vi "read write configuration.vi"(7 "Enum":enum16{"Read", "Write"}(ring)=enum."Write", 8 "error in":errorcluster, 11 "Consumer Cluster in":T1={"This VI Ref"=refnum, "Test VI"=refnum, "Q Ref"=refnum, "UE"=refnum, "Data"=variant, "Timeout"=-1, "Path List[]"=[], "Status"="", "Counter"=0, "Config"={"Source Path"=path "", "Dest Path"=path "", "Log Path"=path "", "Move?"=FALSE, "Log?"=FALSE, "Scanners"=[], "Excude Folders"=[], "Jpg?"=FALSE, "Default path"=path "", "Extended?"=FALSE, "Mode"=enum."Move"}, "Total"=0, "Config Path"=path "", "exif info"={"Make"="Canon\u0000", "Model"="Canon PowerShot A495\u0000", "Orientation"=0, "Date"=timestamp(0 s since 1904-01-01), "Width"=0, "Height"=0, "Square?"=FALSE, "File Name"="Canon\u0000", "Extension"="Canon\u0000", "Valid?"=FALSE, "Path"=path "", "size"=0, "No Ext?"=FALSE, "prefix?"=FALSE, "String"="", "Name Type"=enum."Event Sufix"}, "app operation"=enum."Start", "Log Ref"=refnum, "Start Time"=0.0, "Pause Time"=0.0, "Argument?"=FALSE, "Argument path"=path "", "Identical"=FALSE, "File.lvclass"=refnum}) -> (0 "error out":errorcluster, 3 "cluster out":T1={"This VI Ref"=refnum, "Test VI"=refnum, "Q Ref"=refnum, "UE"=refnum, "Data"=variant, "Timeout"=-1, "Path List[]"=[], "Status"="", "Counter"=0, "Config"={"Source Path"=path "", "Dest Path"=path "", "Log Path"=path "", "Move?"=FALSE, "Log?"=FALSE, "Scanners"=[], "Excude Folders"=[], "Jpg?"=FALSE, "Default path"=path "", "Extended?"=FALSE, "Mode"=enum."Move"}, "Total"=0, "Config Path"=path "", "exif info"={"Make"="Canon\u0000", "Model"="Canon PowerShot A495\u0000", "Orientation"=0, "Date"=timestamp(0 s since 1904-01-01), "Width"=0, "Height"=0, "Square?"=FALSE, "File Name"="Canon\u0000", "Extension"="Canon\u0000", "Valid?"=FALSE, "Path"=path "", "size"=0, "No Ext?"=FALSE, "prefix?"=FALSE, "String"="", "Name Type"=enum."Event Sufix"}, "app operation"=enum."Start", "Log Ref"=refnum, "Start Time"=0.0, "Pause Time"=0.0, "Argument?"=FALSE, "Argument path"=path "", "Identical"=FALSE, "File.lvclass"=refnum})   [LabVIEW 2023, in "User Interface.lvlib"]
uses:
  User Interface.lvlib
  Controls/main consumer cluster.ctl
  File Classes/File/File.lvclass
  Controls/configuration cluster.ctl
  File Classes/Controls/exif data cluster.ctl
  File Classes/Controls/rename type enum.ctl
  Controls/app operation state enum.ctl
  File Classes/File Classes.lvlib
panel:
  # "Output Indicators"
  # "Input Controls"
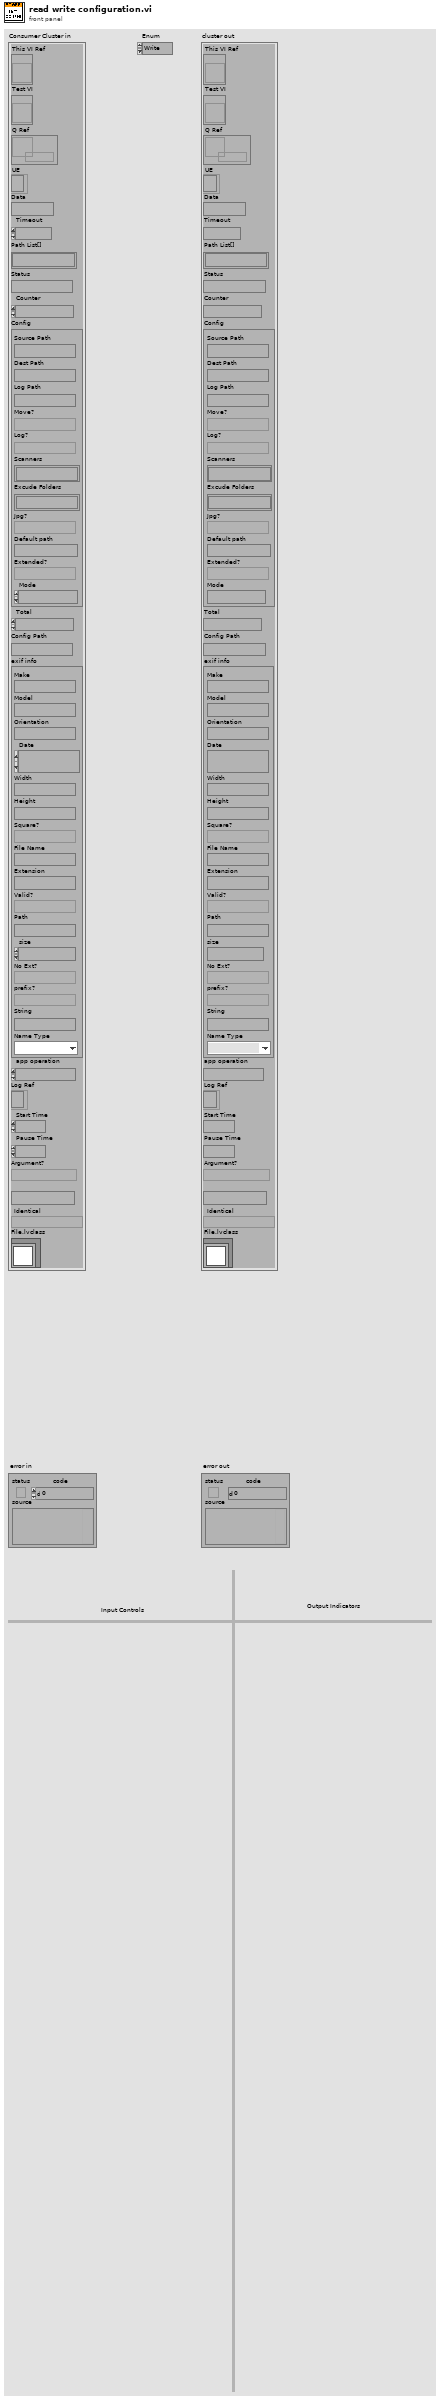
[diagram p1: front panel]
types:
  T1 = typedef "User Interface.lvlib/main consumer cluster.ctl" = cluster{"This VI Ref":refnum<vi>, "Test VI":refnum<vi>, "Q Ref":refnum<queue>, "UE":refnum<event-registration>, "Data":variant, "Timeout":i32, "Path List[]":path[], "Status":string, "Counter":i32, "Config":T2, "Total":i32, "Config Path":path, "exif info":T3, "app operation":T5, "Log Ref":refnum<file>, "Start Time":dbl, "Pause Time":dbl, "Argument?":bool, "Argument path":path, "Identical":bool, "File.lvclass":refnum<class "File.lvclass">}
  T2 = typedef "User Interface.lvlib/configuration cluster.ctl" = cluster{"Source Path":path, "Dest Path":path, "Log Path":path, "Move?":bool, "Log?":bool, "Scanners":string[], "Excude Folders":string[], "Jpg?":bool, "Default path":path, "Extended?":bool, "Mode":enum16{"Copy (Default)", "Move", "Rename"}}
  T3 = typedef "File Classes.lvlib/exif data cluster.ctl" = cluster{"Make":string, "Model":string, "Orientation":u16, "Date":timestamp, "Width":u16, "Height":u16, "Square?":bool, "File Name":string, "Extension":string, "Valid?":bool, "Path":path, "size":i64, "No Ext?":bool, "prefix?":bool, "String":string, "Name Type":T4}
  T4 = typedef "File Classes.lvlib/rename type enum.ctl" = enum16{"Date & Time (Default)", "Model Sufix", "Event Sufix", "Model & Event Sufix"}
  T5 = typedef "User Interface.lvlib/app operation state enum.ctl" = enum16{"Start", "Stop", "Pause", "Resume"}
  T6 = enum16{"open", "replace", "create", "open or create", "replace or create", "replace or create with confirmation"}
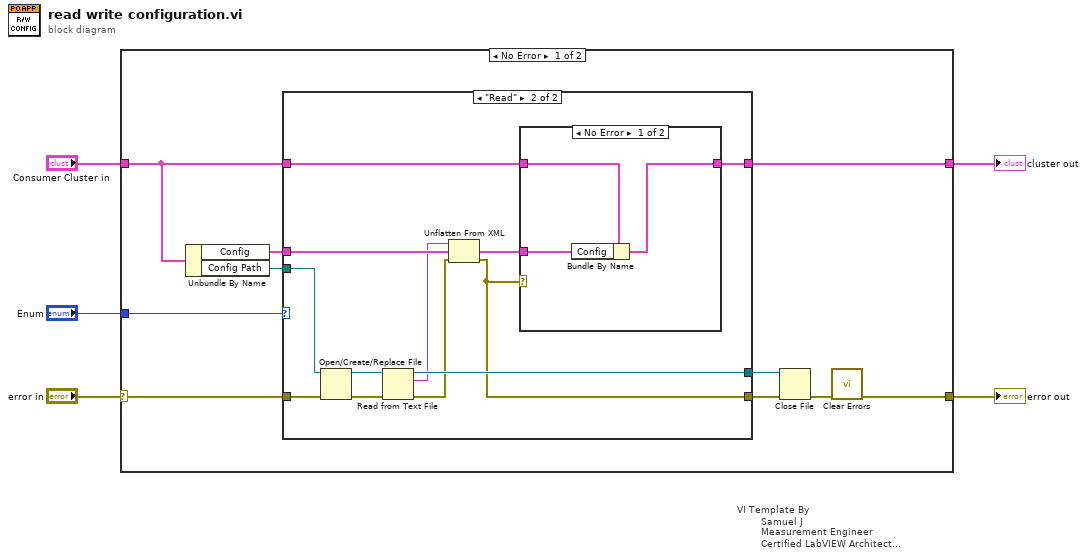
[diagram p0: block diagram]
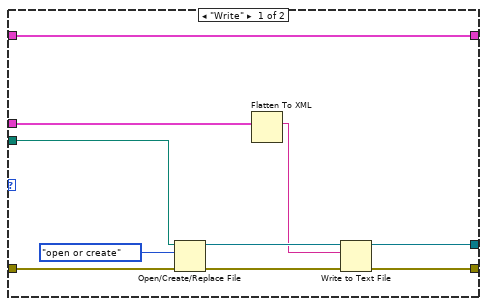
[diagram p2: hidden frame]
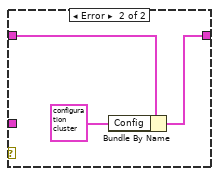
[diagram p3: hidden frame]
diagram:
  n1 = case "VI Template By\n        Samuel J\n        Measurement Engineer\n        Certified LabVIEW Architect\n        Vestas Technology R&D Chennai" shown="No Error" "error in" {
    selector: "error in" -> [w12 w45]
    tunnel: [w6 w45] -> w4
    tunnel: [w10 w44] -> w2
    tunnel: "Consumer Cluster in" -> [w9 w44]
    tunnel: "Enum" -> [w7 _]
    frame No Error {
      n2 = Unbundle By Name(w9) -> ("Config"=w13:T2, "Config Path"=w8:path)
      n3 = case shown="\"Read\"" w7 {
        tunnel: [w24 w36] -> w15
        tunnel: [w22 w26] -> w14
        tunnel: w13 -> [w21 w32]
        tunnel: w12 -> [w19 w34]
        tunnel: [w18 w28] -> w10
        tunnel: w9 -> [w18 w29]
        tunnel: w8 -> [w16 w33]
        frame "Write" {
          n4 = Open/Create/Replace File(file path (use dialog)=w16, error in=w19, operation (0:open)=T6."open or create") -> (refnum out=w25:refnum<file>, error out=w23:errorcluster)  [unwired: 3 in, 1 out]
          n5 = Flatten To XML(6:w21) -> (2:w20:string)
          n6 = Write to Text File(file (use dialog)=w25, text=w20, error in=w23) -> (refnum out=w24:refnum<file>, error out=w22:errorcluster)  [unwired: 1 in, 1 out]
        }
        frame "Read" {
          n7 = Open/Create/Replace File(file path (use dialog)=w33, error in=w34) -> (refnum out=w37:refnum<file>, error out=w35:errorcluster)  [unwired: 4 in, 1 out]
          n8 = Read from Text File(file (use dialog)=w37, error in=w35) -> (refnum out=w36:refnum<file>, text=w31:string, error out=w30:errorcluster)  [unwired: 2 in, 1 out]
          n9 = Unflatten From XML(xml string=w31, type=w32, error in (no error)=w30) -> (value=w27:T2, error out=w26:errorcluster)
          n10 = case shown="No Error" w26 {
            tunnel: w29 -> [w40 w43]
            tunnel: [w39 w42] -> w28
            tunnel: w27 -> [w38 _]
            frame No Error {
              n11 = Bundle By Name(cluster=w40, "Config"=w38) -> (w39:T1)
            }
            frame Error {
              n12 = Bundle By Name(cluster=w43, "Config"=T2 {"Source Path"=path "", "Dest Path"=path "", "Log Path"=path "", "Move?"=FALSE, "Log?"=TRUE, "Scanners"=[], "Excude Folders"=[], "Jpg?"=FALSE, "Default path"=path "", "Extended?"=FALSE, "Mode"=enum."Move"}) -> (w42:T1)
            }
          }
        }
      }
      n13 = Close File(refnum=w15, error in=w14) -> (error out=w11:errorcluster)  [unwired: 1 out]
      n14 = call <vilib>:"Clear Errors.vi"("error in (no error)"=w11) -> ("error out"=w6:errorcluster)  [unwired: 5 in, 1 out]
    }
    frame Error {
    }
  }
  "error out" <- w4
  "cluster out" <- w2
